vi "Ballard - Arinc-429 - Add All Label Bit Channels.vi"(8 "error in (no error)":errorcluster, 11 "Node Ptr":u64 format="%.0x") -> (0 "error out":errorcluster)   [LabVIEW 2016, in "Ballard Arinc-429 System Explorer.lvlib"]
uses:
  Ballard Arinc-429 System Explorer.lvlib
  Shared/Controls and Global/Global.vi
  Shared/Ballard Arinc-429 Shared.lvlib
  <vilib>/NI Veristand/Custom Device API/Custom Device Channel Type.ctl
  <vilib>/NI VeriStand/Custom Device API/Custom Device API.lvlib
  <vilib>/NI Veristand/Custom Device API/Custom Device Channel.ctl
  <vilib>/NI Veristand/Custom Device API/Get Item Property (U32).vi
  Shared/Controls and Global/Number of Bits.ctl
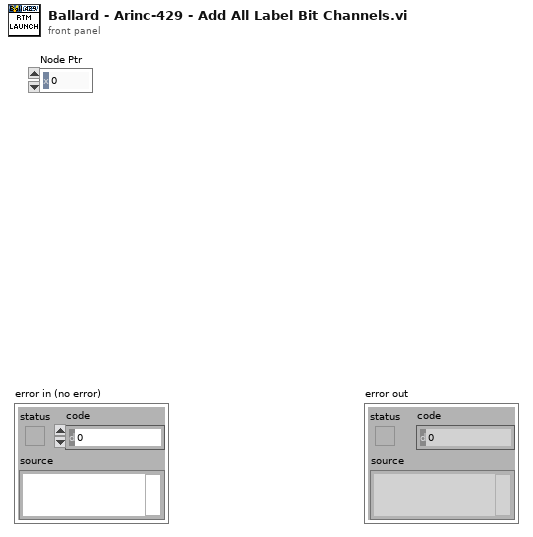
[diagram p1: front panel]
types:
  T1 = typedef "Custom Device API.lvlib/Custom Device Channel Type.ctl" = enum16{"Input", "Output"}
  T2 = typedef "Custom Device API.lvlib/Custom Device Channel.ctl" = cluster{"Type":T1, "Units":string, "Default Value":dbl, "Faultable":bool, "Scalable":bool}
  T3 = typedef "Custom Device API.lvlib/Custom Device Item Ref.ctl" = u64
  T4 = typedef "Ballard Arinc-429 Shared.lvlib/Number of Bits.ctl" = i32
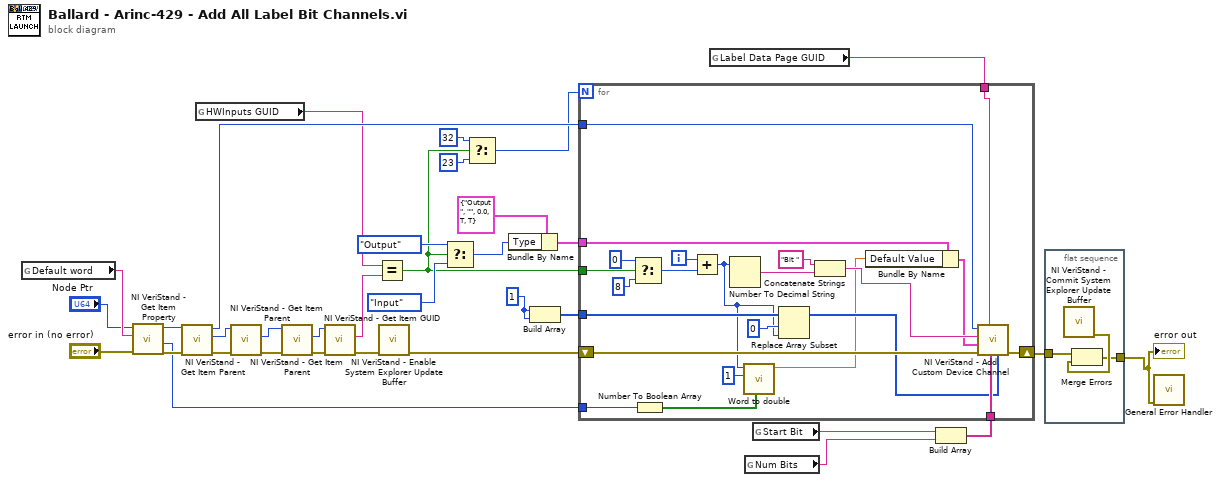
[diagram p0: block diagram]
diagram:
  w20 = 1 ("element")
  n1 = global read "Global.vi" "Default word"() -> (w12:string)
  n2 = call-poly <vilib>:"NI VeriStand - Get Item Property.vi"("error in (no error)"="error in (no error)", "Property Name"=w12, "Item Ref in"="Node Ptr") -> ("error out"=w8:errorcluster, "Value"=w7:u32, "Item Ref out"=w9:T3)  [unwired: 5 in, 1 out]
  n3 = call <vilib>:"NI VeriStand - Get Item Parent.vi"("error in (no error)"=w8, "Item Ref in"=w9) -> ("error out"=w23:errorcluster, "Parent Ref"=w24:T3, "Item Ref out"=w32:T3)  [unwired: 6 in, 1 out]
  n4 = global read "Global.vi" "HWInputs GUID"() -> (w30:string)
  n5 = call <vilib>:"NI VeriStand - Get Item Parent.vi"("error in (no error)"=w23, "Item Ref in"=w24) -> ("error out"=w4:errorcluster, "Parent Ref"=w2:T3)  [unwired: 6 in, 2 out]
  n6 = call <vilib>:"NI VeriStand - Get Item Parent.vi"("error in (no error)"=w4, "Item Ref in"=w2) -> ("error out"=w3:errorcluster, "Parent Ref"=w1:T3)  [unwired: 6 in, 2 out]
  n7 = call <vilib>:"NI VeriStand - Get Item GUID.vi"("error in (no error)"=w3, "Item Ref in"=w1) -> ("error out"=w18:errorcluster, "GUID"=w31:string)  [unwired: 7 in, 1 out]
  n8 = Equal?(x=w30, y=w31) -> (x = y?=w13:bool)
  n9 = call <vilib>:"NI VeriStand - Enable System Explorer Update Buffer.vi"("error in (no error)"=w18) -> ("error out"=w17:errorcluster)  [unwired: 10 in]
  n10 = Select(t=Custom_Device_Channel_Type."Output" ("Type"), s=w13, f=Custom_Device_Channel_Type."Input" ("Type")) -> (s? t:f=w27:T1)
  n11 = Select(t=32, s=w13, f=23) -> (s? t:f=w15:i32)
  n12 = Bundle By Name(cluster=T2 {"Type"=enum."Output", "Units"="", "Default Value"=0.0, "Faultable"=TRUE, "Scalable"=TRUE} ("Channel"), "Type"=w27) -> (w25:T2)
  n13 = Build Array(w20, w20) -> (w19:i32[])
  n14 = global read "Global.vi" "Label Data Page GUID"() -> (w22:string)
  n15 = global read "Global.vi" "Num Bits"() -> (w21:string)
  n16 = global read "Global.vi" "Start Bit"() -> (w34:string)
  n17 = Build Array(w34, w21) -> (w33:string[])
  n18 = for {
    N: w15 -> [_]
    shift-right: [w53] -> w6
    shift-left: w17 -> [w57]
    tunnel: w32 -> [w51]
    tunnel: w33 -> [w52]
    tunnel: w25 -> [w50]
    tunnel: w22 -> [w49]
    tunnel: w19 -> [w48]
    tunnel: w13 -> [w43]
    tunnel: w7 -> [w36]
    i -> [w47]
    n19 = Select(t=0 ("y"), s=w43, f=8 ("y")) -> (s? t:f=w44:i32)
    n20 = Number To Boolean Array(number=w36) -> (Boolean array=w35:bool[])
    n21 = Add(x=w47, y=w44) -> (x+y=w40:i32)
    n22 = Number To Decimal String(number=w40) -> (decimal integer string=w55:string)  [unwired: 1 in]
    n23 = call "Word to double.vi"("Word"=w35, "Number of Bits"=T4 1, "Start Bit"=w40) -> ("Double"=w37:dbl)  [unwired: 8 in]
    n24 = Replace Array Subset(array=w48, new element=w40, index=0) -> (w46:i32[])
    n25 = Concatenate Strings("Bit " ("string"), w55) -> (w54:string)
    n26 = Bundle By Name(cluster=w50, "Default Value"=w37) -> (w38:T2)
    n27 = call <vilib>:"NI VeriStand - Add Custom Device Channel.vi"("Property Values"=w46, "Property names"=w52, "GUID (Default Channel)"=w49, "error in (no error)"=w57, "Channel"=w38, "Channel Name"=w54, "Parent Ref in"=w51) -> ("error out"=w53:errorcluster)  [unwired: 1 in, 3 out]
  }
  n28 = flat-sequence {
    tunnel: w6 -> [w60]
    tunnel: [w58] -> w5
    frame #0 {
      n29 = call <vilib>:"NI VeriStand - Commit System Explorer Update Buffer.vi"() -> ("error out"=w59:errorcluster)  [unwired: 11 in]
      n30 = Merge Errors(w60, w59) -> (w58:errorcluster)
    }
  }
  n31 = call <vilib>:"General Error Handler.vi"("error in (no error)"=w5) -> ()  [unwired: 10 in, 5 out]
  "error out" <- w5
